vi "oa_Generate Waveform Reference with Vector Reference (1 Channel).vi"(0 "resampled signal":cluster{"r0":dbl, "dr":dbl, "Y":dbl[]}={"r0"=0.0, "dr"=1.0, "Y"=[]} {"r0" format="%.2p"; "dr" format="%.2p"; "Y" format="%.2f"}, 1 "reset? (True)":bool=TRUE, 5 "slow roll vectors":cdb[](array[numeric]) format="%.2f", 7 "orders to compensate":dbl[](array[numeric])=[1.0] format="%.2f", 9 "interpolated pulse positions":dbl[](array[numeric]) format="%.2f", 11 "error out in":errorcluster) -> (4 "resampled signal out":cluster{"r0":dbl, "dr":dbl, "Y":dbl[]}={"r0"=0.0, "dr"=1.0, "Y"=[]} {"r0" format="%.2p"; "dr" format="%.2p"; "Y" format="%.2f"}, 6 "baseline in":cluster{"r0":dbl, "dr":dbl, "Y":dbl[]}={"r0"=0.0, "dr"=1.0, "Y"=[]} {"r0" format="%.2p"; "dr" format="%.2p"; "Y" format="%.2f"}, 8 "slow roll vectors out":cdb[](array[numeric]) format="%.2f", 15 "error out":errorcluster)   [LabVIEW 2017, in "SoundVib_RefDataProcess.lvlib"]
uses:
  <vilib>/addons/Sound and Vibration/Order Analysis/Referece Data Processing/SoundVib_RefDataProcess.lvlib
  <vilib>/Analysis/NI_AALBase.lvlib
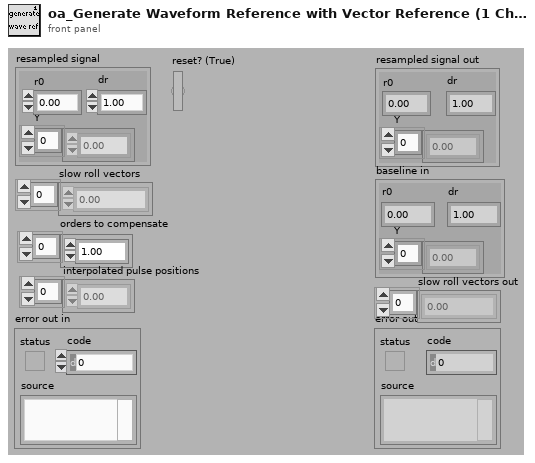
[diagram p1: front panel]
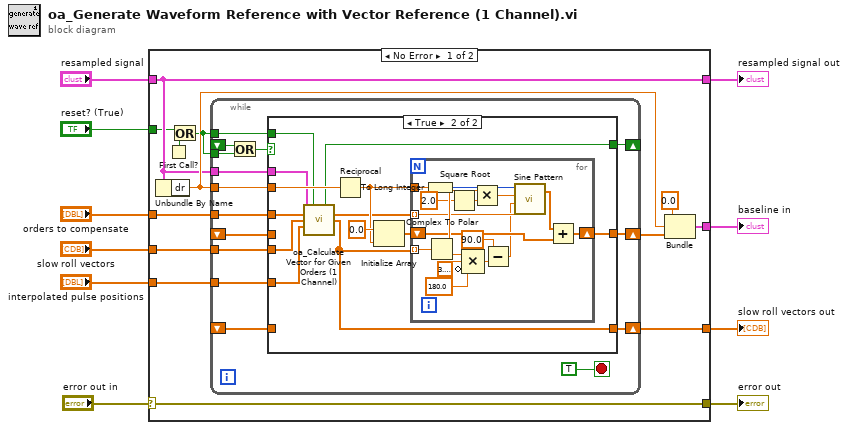
[diagram p0: block diagram]
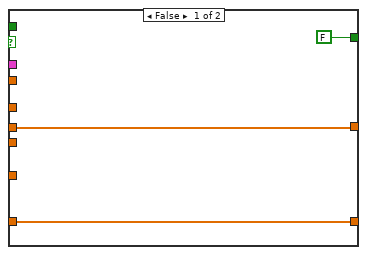
[diagram p2: hidden frame]
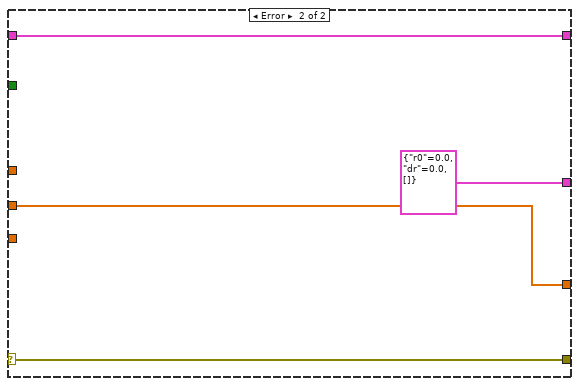
[diagram p3: hidden frame]
diagram:
  n1 = case shown="No Error" "error out in" {
    selector: "error out in" -> [w17 w75]
    tunnel: [w17 w75] -> w9
    tunnel: "reset? (True)" -> [w13 _]
    tunnel: "resampled signal" -> [w16 w74]
    tunnel: [w16 w74] -> w6
    tunnel: "orders to compensate" -> [w23 _]
    tunnel: "slow roll vectors" -> [w22 w72]
    tunnel: [w18 cluster{"r0":dbl, "dr":dbl, dbl[]} {"r0"=0.0, "dr"=0.0, []}] -> w3
    tunnel: "interpolated pulse positions" -> [w15 _]
    tunnel: [w14 w72] -> w1
    frame No Error {
      n2 = Unbundle By Name(w16) -> ("dr"=w20:dbl)
      n3 = First Call?() -> (First Call?: T/F=w11:bool)
      n4 = Or(x=w13, y=w11) -> (x .or. y?=w12:bool)
      n5 = while {
        tunnel: w12 -> [w25]
        tunnel: w23 -> [w38]
        tunnel: w22 -> [w37]
        tunnel: w20 -> [w36]
        shift-right: [w34] -> w21
        shift-left: _ -> [w33]
        tunnel: w16 -> [w32]
        tunnel: w15 -> [w31]
        shift-right: [w30] -> w14
        shift-left: _ -> [w29]
        tunnel: w12 -> [w28]
        shift-right: [w27] -> _
        shift-left: _ -> [w26]
        stop <- TRUE stop-if-true
        n6 = Or(x=w26, y=w25) -> (x .or. y?=w24:bool)
        n7 = case shown="True" w24 {
          tunnel: w38 -> [_ w48]
          tunnel: w37 -> [_ w47]
          tunnel: w36 -> [_ w54]
          tunnel: [w41 w50] -> w34
          tunnel: w33 -> [w41 _]
          tunnel: w32 -> [_ w49]
          tunnel: w31 -> [_ w46]
          tunnel: [w40 w44] -> w30
          tunnel: w29 -> [w40 _]
          tunnel: w28 -> [_ w43]
          tunnel: [FALSE ("reset out") w42] -> w27
          frame False {
          }
          frame True {
            n8 = call <vilib>:"oa_Calculate Vector for Given Orders (1 Channel).vi"("resampled signal"=w49, "reset? (True)"=w43, "orders to compensate"=w48, "slow roll vectors"=w47, "interpolated pulse positions"=w46) -> ("reset out"=w42:bool, "orders out"=w45:dbl[], "slow roll vectors out"=w44:cdb[])  [unwired: 7 in, 1 out]
            n9 = Reciprocal(x=w54) -> (1/x=w52:dbl)
            n10 = Initialize Array(0.0 ("element"), w52) -> (w51:dbl[])
            n11 = for {
              tunnel: w45 -> [w67] mode=indexing
              tunnel: w44 -> [w71] mode=indexing
              tunnel: w52 -> [w70]
              shift-right: [w65] -> w50
              shift-left: w51 -> [w64]
              n12 = To Long Integer(number=w70) -> (32bit integer=w69:i32)
              n13 = Complex To Polar(r * e^(i*theta)=w71) -> (r=w68:dbl, theta=w63:dbl)
              n14 = Square Root(x=2.0) -> (sqrt(x)=w56:dbl)
              n15 = Compound Arithmetic op=MULTIPLY(w63, 3.141592653589793, invert 180.0 ("value")) -> (w60:dbl)
              n16 = Multiply(x=w68, y=w56) -> (x*y=w57:dbl)
              n17 = Subtract(x=90.0, y=w60) -> (x-y=w58:dbl)
              n18 = call <vilib>:"Sine Pattern.vi"("cycles"=w67, "phase(degrees)"=w58, "amplitude"=w57, "samples"=w69) -> ("Sinusoidal Pattern"=w66:dbl[])  [unwired: 1 out]
              n19 = Add(x=w66, y=w64) -> (x+y=w65:dbl[])
            }
          }
        }
      }
      n20 = Bundle("r0"=0.0, "dr"=w20, w21) -> (w18:cluster{"r0":dbl, "dr":dbl, dbl[]})  [unwired: 1 in]
    }
    frame Error {
    }
  }
  "error out" <- w9
  "resampled signal out" <- w6
  "baseline in" <- w3
  "slow roll vectors out" <- w1
